vi "Loop_HW.vi"   [LabVIEW 2017, in "Controller.lvlib"]
uses:
  Controller.lvlib
  Globals/Global_HW_Address_Assignments.vi
  _SHARE ALL/Global Share All/Global_STOP.vi
  Global_Data Out.vi
types:
  T1 = typedef "WPI_JoystickDeviceEnum.ctl" = enum16{"USB 0", "USB 1", "USB 2", "USB 3", "USB 4", "USB 5"}
  T2 = typedef "WPI_JoystickDevRef.ctl" = cluster{"Device":T1}
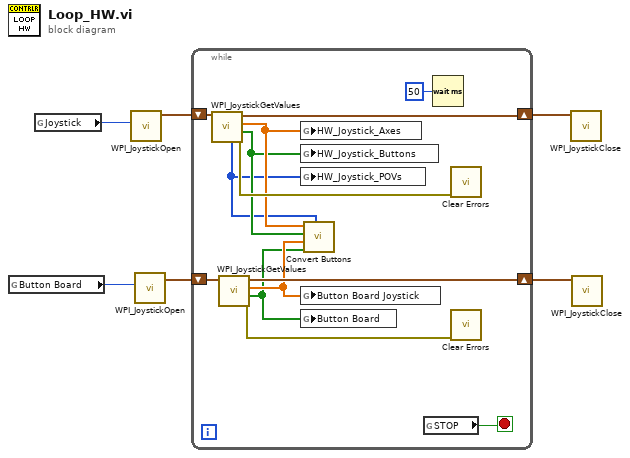
[diagram p0: block diagram]
diagram:
  n1 = global read "Global_HW_Address_Assignments.vi" "Button Board"() -> (w2:T1)
  n2 = global read "Global_HW_Address_Assignments.vi" "Joystick"() -> (w1:T1)
  n3 = call <vilib>:"WPI_JoystickOpen.vi"("JoystickDevice"=w1) -> ("JoystickDevRef"=w5:T2)  [unwired: 10 in]
  n4 = call <vilib>:"WPI_JoystickOpen.vi"("JoystickDevice"=w2) -> ("JoystickDevRef"=w4:T2)  [unwired: 10 in]
  n5 = while {
    shift-right: [w18] -> w6
    shift-left: w5 -> [w19]
    shift-right: [w10] -> w3
    shift-left: w4 -> [w13]
    stop <- w17 stop-if-true
    n6 = call <vilib>:"WPI_JoystickGetValues.vi"("JoystickDevRef"=w19) -> ("error out"=w15:errorcluster, "Buttons"=w11:bool[], "Axes"=w12:dbl[], "JoystickDevRef"=w18:T2, "POVs"=w7:i16[])  [unwired: 6 in]
    n7 = call <vilib>:"WPI_JoystickGetValues.vi"("JoystickDevRef"=w13) -> ("error out"=w14:errorcluster, "Buttons"=w8:bool[], "Axes"=w9:dbl[], "JoystickDevRef"=w10:T2)  [unwired: 6 in, 1 out]
    n8 = global write "Global_Data Out.vi" "HW_Joystick_Axes"(w12) -> ()
    n9 = global write "Global_Data Out.vi" "HW_Joystick_Buttons"(w11) -> ()
    n10 = global write "Global_Data Out.vi" "HW_Joystick_POVs"(w7) -> ()
    n11 = global write "Global_Data Out.vi" "Button Board Joystick"(w9) -> ()
    n12 = global write "Global_Data Out.vi" "Button Board"(w8) -> ()
    n13 = call "Convert Buttons.vi"("POVs"=w7, "HW_Button Board"=w8, "HW_Button Board_Axes"=w9, "HW_Joystick_Buttons"=w11, "HW_Joystick_Axes"=w12) -> ()  [unwired: 7 in]
    n14 = global read "Global_STOP.vi" "STOP"() -> (w17:bool)
    n15 = Wait (ms)(milliseconds to wait=u32 50) -> ()  [unwired: 1 out]
    n16 = call <vilib>:"Clear Errors.vi"("error in (no error)"=w15) -> ()  [unwired: 5 in, 2 out]
    n17 = call <vilib>:"Clear Errors.vi"("error in (no error)"=w14) -> ()  [unwired: 5 in, 2 out]
  }
  n18 = call <vilib>:"WPI_JoystickClose.vi"("JoystickDevRef"=w6) -> ()  [unwired: 11 in]
  n19 = call <vilib>:"WPI_JoystickClose.vi"("JoystickDevRef"=w3) -> ()  [unwired: 11 in]
